vi "GeneratorChangeFrequency.vi"(9 "GeneratorChangeFreq":dbl, 10 "GEN error":errorcluster, 11 "GEN VISA":refnum<visa-resource-name>) -> (2 "error out":errorcluster, 3 "VISA resource name out":refnum<visa-resource-name>)   [LabVIEW 2021]
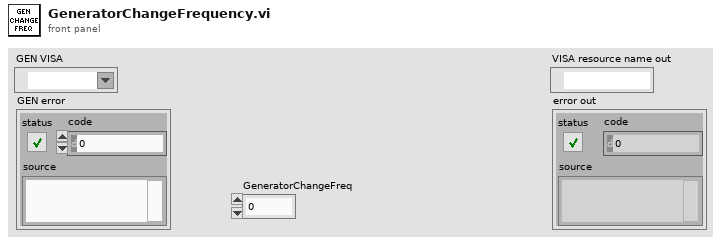
[diagram p1: front panel]
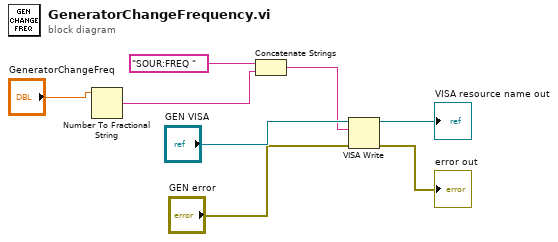
[diagram p0: block diagram]
diagram:
  n1 = Number To Fractional String(number="GeneratorChangeFreq") -> (F-format string=w4:string)  [unwired: 3 in]
  n2 = Concatenate Strings("SOUR:FREQ ", w4) -> (w3:string)
  n3 = VISA Write(VISA resource name="GEN VISA", write buffer=w3, error in (no error)="GEN error") -> (VISA resource name out=→"VISA resource name out":refnum<visa-resource-name>, error out=→"error out":errorcluster)  [unwired: 1 out]
